vi "Monitor.vi"(8 "error in (no error)":errorcluster, 10 "Numeric":i8, 11 "VISA resource name":refnum<visa-resource-name>) -> (0 "error out 2":errorcluster, 1 "read buffer":string, 2 "concatenated string":string, 3 "VISA resource name out":refnum<visa-resource-name>)   [LabVIEW 2012, in "Fluke 2625A.lvlib"]
uses:
  <instrlib>/Fluke 2625A/Fluke 2625A.lvlib
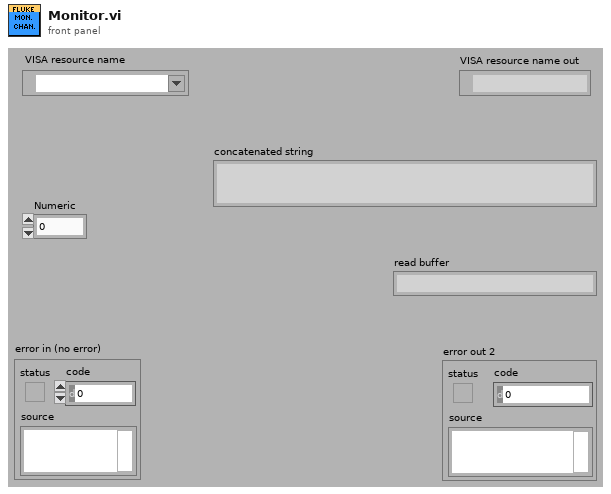
[diagram p1: front panel]
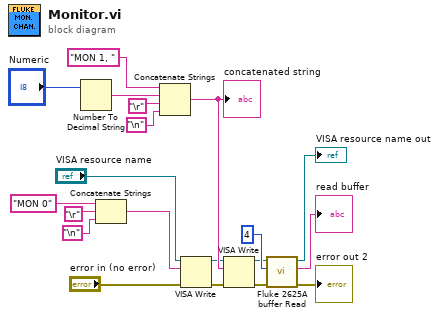
[diagram p0: block diagram]
diagram:
  n1 = Number To Decimal String(number="Numeric") -> (decimal integer string=w11:string)  [unwired: 1 in]
  n2 = Concatenate Strings("MON 0" ("write buffer"), "\r", "\n") -> (w4:string)
  n3 = Concatenate Strings("MON 1, " ("string"), w11, "\r", "\n") -> (w14:string)
  "concatenated string" <- w14
  n4 = VISA Write(VISA resource name="VISA resource name", write buffer=w4, error in (no error)="error in (no error)") -> (VISA resource name out=w6:refnum<visa-resource-name>, error out=w5:errorcluster)  [unwired: 1 out]
  n5 = VISA Write(VISA resource name=w6, write buffer=w14, error in (no error)=w5) -> (VISA resource name out=w15:refnum<visa-resource-name>, error out=w16:errorcluster)  [unwired: 1 out]
  n6 = call <instrlib>:"Fluke 2625A buffer Read.vi"("error out"=w16, "byte count"=u32 4, "VISA resource name out"=w15) -> ("error out 2"=→"error out 2":errorcluster, "read buffer"=→"read buffer":string, "VISA resource name out 2"=→"VISA resource name out":refnum<visa-resource-name>)  [unwired: 5 in, 1 out]
